vi "CTRE_Phoenix_MotorControl_ConfigPeakOutput.vi"(6 "timeoutMs":u32, 8 "error in (no error)":errorcluster, 9 "Reverse Peak Percent Output":dbl, 10 "Forward Peak Percent Output":dbl, 11 "CAN Talon SRX Ref":T1={"DeviceStatus"={"status"=FALSE, "code"=0, "source"=""}, "Type"=enum."PWM", "PWM"={"PWM Channel"=enum."PWM 1", "DeadBand"={"Name"="", "maxPositivePwm"=0, "minPositivePwm"=0, "centerPwm"=0, "maxNegativePwm"=0, "minNegativePwm"=0, "angularRange"=0}}, "CAN"={"Device Number"=0, "SetOutput VI Ref"=variant(enum8{"Percent VBus", "Current", "Speed", "Position", "Voltage"} enum."Percent VBus"), "GetOutput VI Ref"=variant(refnum<k1> refnum), "Enable VI Ref"=variant(dbl 12.0), "Disable VI Ref"=variant(enum8{"Percent VBus", "Speed", "Position", "Slave", "Unchanged / Invalid", "Voltage Compensation", "Current", "Motion Profile"} enum."Percent VBus"), "Data"=variant}, "Invert"=FALSE, "DIO PWM"={"PWM \"Enable\" Channel"=enum."Invalid", "DIOChannel"=enum."Invalid", "PWM Rate"=0.0}}) -> (0 "error out":errorcluster, 3 "CAN Talon SRX Ref":T1={"DeviceStatus"={"status"=FALSE, "code"=0, "source"=""}, "Type"=enum."PWM", "PWM"={"PWM Channel"=enum."PWM 1", "DeadBand"={"Name"="", "maxPositivePwm"=0, "minPositivePwm"=0, "centerPwm"=0, "maxNegativePwm"=0, "minNegativePwm"=0, "angularRange"=0}}, "CAN"={"Device Number"=0, "SetOutput VI Ref"=variant(enum8{"Percent VBus", "Current", "Speed", "Position", "Voltage"} enum."Percent VBus"), "GetOutput VI Ref"=variant(refnum<k1> refnum), "Enable VI Ref"=variant(dbl 12.0), "Disable VI Ref"=variant(enum8{"Percent VBus", "Speed", "Position", "Slave", "Unchanged / Invalid", "Voltage Compensation", "Current", "Motion Profile"} enum."Percent VBus"), "Data"=variant}, "Invert"=FALSE, "DIO PWM"={"PWM \"Enable\" Channel"=enum."Invalid", "DIOChannel"=enum."Invalid", "PWM Rate"=0.0}})   [LabVIEW 2017]
doc: "Configures the Peak (maximum) Percent Output in the forward and reverse directions. Peak values apply in all control modes."
uses:
  <vilib>/Rock Robotics/WPI/MotorControl/WPI_MotorControlDeviceRef.ctl
  <vilib>/Rock Robotics/WPI/MotorControl/WPI_MotorControlType.ctl
  <vilib>/Rock Robotics/SystemInterfaces/DIO/FPGA_DIOPWMChannel.ctl
  <vilib>/Rock Robotics/WPI/PWM/WPI_PWMDeadband.ctl
  <vilib>/Rock Robotics/SystemInterfaces/DIO/FPGA_DIOChannel.ctl
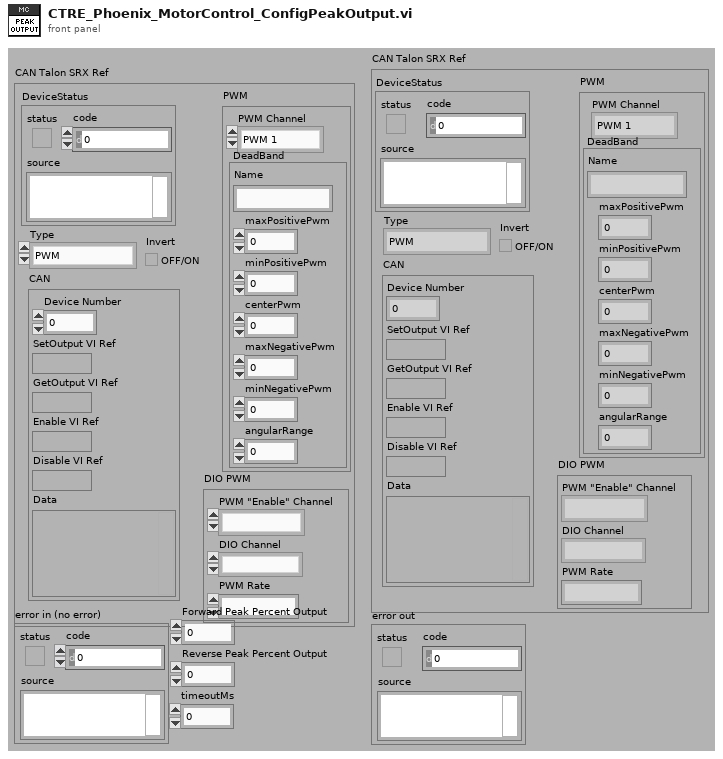
[diagram p1: front panel]
types:
  T1 = typedef "WPI_MotorControlDeviceRef.ctl" = cluster{"DeviceStatus":errorcluster, "Type":T2, "PWM":cluster{"PWM Channel":T3, "DeadBand":T4}, "CAN":cluster{"Device Number":u8, "SetOutput VI Ref":variant, "GetOutput VI Ref":variant, "Enable VI Ref":variant, "Disable VI Ref":variant, "Data":variant}, "Invert":bool, "DIO PWM":cluster{"PWM \"Enable\" Channel":T3, "DIOChannel":T5, "PWM Rate":dbl}}
  T2 = typedef "WPI_MotorControlType.ctl" = enum16{"PWM", "CAN", "DIO PWM"}
  T3 = typedef "FPGA_DIOPWMChannel.ctl" = enum8{"PWM 0", "PWM 1", "PWM 2", "PWM 3", "PWM 4", "PWM 5", "PWM 6", "PWM 7", "PWM 8", "PWM 9", "PWM MXP 0", "PWM MXP 1", "PWM MXP 2", "PWM MXP 3", "PWM MXP 4", "PWM MXP 5", "PWM MXP 6", "PWM MXP 7", "PWM MXP 8", "PWM MXP 9", "Invalid"}
  T4 = typedef "WPI_PWMDeadband.ctl" = cluster{"Name":string, "maxPositivePwm":i32, "minPositivePwm":i32, "centerPwm":i32, "maxNegativePwm":i32, "minNegativePwm":i32, "angularRange":u16}
  T5 = typedef "FPGA_DIOChannel.ctl" = enum8{"DIO 0", "DIO 1", "DIO 2", "DIO 3", "DIO 4", "DIO 5", "DIO 6", "DIO 7", "DIO 8", "DIO 9", "DIO MXP 0", "DIO MXP 1", "DIO MXP 2", "DIO MXP 3", "DIO MXP 4", "DIO MXP 5", "DIO MXP 6", "DIO MXP 7", "DIO MXP 8", "DIO MXP 9", "DIO MXP 10", "DIO MXP 11", "DIO MXP 12", "DIO MXP 13", "DIO MXP 14", "DIO MXP 15", "SPI Port CS1", "SPI Port CS2", "SPI Port CS3", "SPI Port MISO", "SPI Port MOSI", "Invalid"}
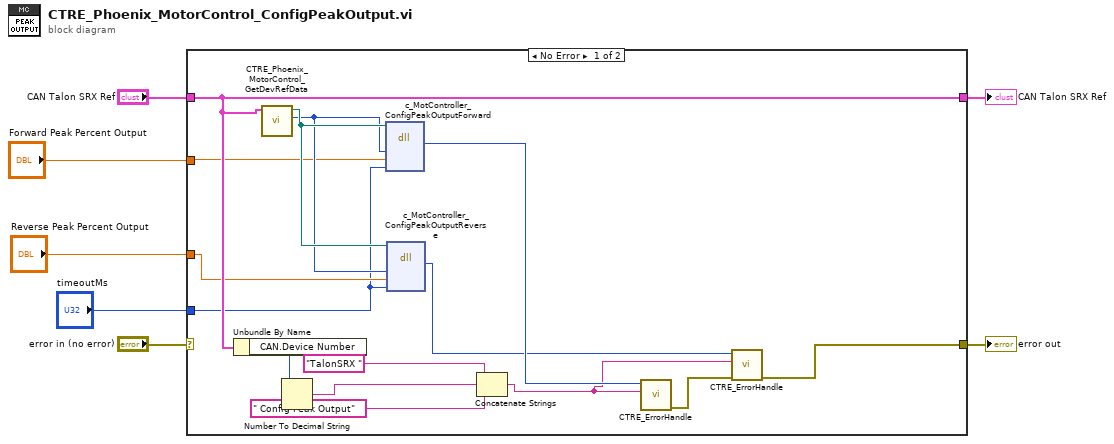
[diagram p0: block diagram]
diagram:
  n1 = case shown="No Error" "error in (no error)" {
    selector: "error in (no error)" -> [_ w24]
    tunnel: [w11 w24] -> w7
    tunnel: "CAN Talon SRX Ref" -> [w18 w23]
    tunnel: [w18 w23] -> w5
    tunnel: "Forward Peak Percent Output" -> [w14 _]
    tunnel: "Reverse Peak Percent Output" -> [w13 _]
    tunnel: "timeoutMs" -> [w8 _]
    frame No Error {
      n2 = Unbundle By Name(w18) -> ("CAN.Device Number"=w19:u8)
      n3 = call "CTRE_Phoenix_MotorControl_GetDevRefData.vi"("MotorControlDevRef"=w18) -> ("handle"=w15:u64, "Library"=w16:path)  [unwired: 4 in, 5 out]
      n4 = Number To Decimal String(number=w19) -> (decimal integer string=w21:string)  [unwired: 1 in]
      n5 = dll-call lib="?" fn="c_MotController_ConfigPeakOutputForward"(path in=w16, "handle"=w15, "percentOut"=w14, "timeoutMs"=w8) -> ("ErrorCode"=w17:i32)  [unwired: 5 in, 2 out]
      n6 = dll-call lib="?" fn="c_MotController_ConfigPeakOutputReverse"(path in=w16, "handle"=w15, "percentOut"=w13, "timeoutMs"=w8) -> ("ErrorCode"=w10:i32)  [unwired: 5 in, 2 out]
      n7 = Concatenate Strings("TalonSRX " ("string"), w21, " Config Peak Output" ("string")) -> (w9:string)
      n8 = call "CTRE_ErrorHandle.vi"("origin"=w9, "code"=w17) -> ("error out"=w12:errorcluster)  [unwired: 9 in]
      n9 = call "CTRE_ErrorHandle.vi"("error in"=w12, "origin"=w9, "code"=w10) -> ("error out"=w11:errorcluster)  [unwired: 8 in]
    }
    frame Error {
    }
  }
  "CAN Talon SRX Ref" <- w5
  "error out" <- w7
